vi "FindAndHighlightPoint.vi"(7 "Data In":T1={"Calibration Input"=[], "CalibrationResults"={"Center in Pixels"=[374.0120339529387, 375.46592887074246], "Angle"=0.022945275255000355, "Pixels/MHz X"=0.0, "Pixels/MHz Y"=0.0}, "Highlight"=[], "Running Script"=refnum}, 8 "error in (no error)":errorcluster, 9 "Vertical":i32, 10 "Horizontal":i32, 11 "Value":i32[][](array[numeric])) -> (0 "error out":errorcluster, 2 "Data Out":T1={"Calibration Input"=[], "CalibrationResults"={"Center in Pixels"=[374.0120339529387, 375.46592887074246], "Angle"=0.022945275255000355, "Pixels/MHz X"=0.0, "Pixels/MHz Y"=0.0}, "Highlight"=[], "Running Script"=refnum}, 3 "Numeric":i32)   [LabVIEW 2017]
uses:
  TypeDefinitions/ExperimentVariables.ctl
  ImageAcquisitionProgram/ImageAcquisitionLibrary/GlobalFrontPanelReferences.vi
  ImageAcquisitionProgram/ImageAcquisitionLibrary/ImageAcquisitionLibrary.lvlib
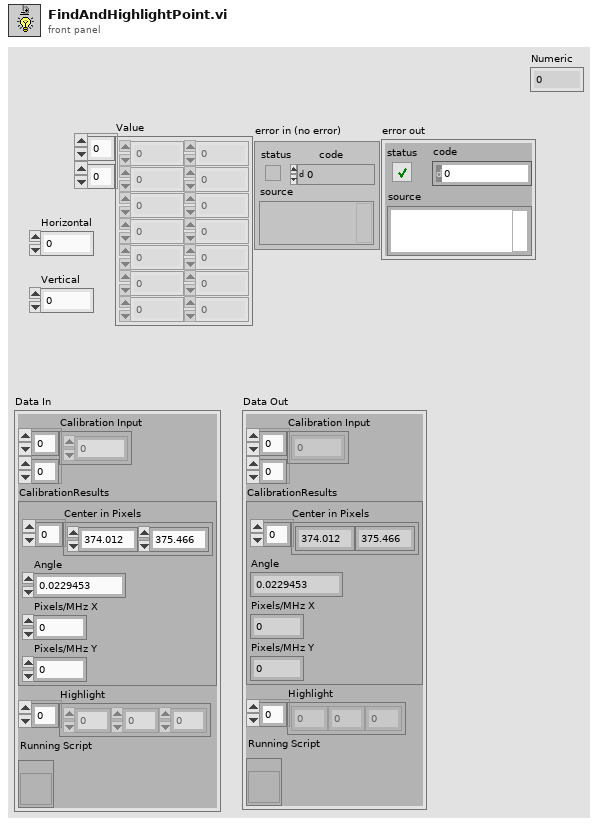
[diagram p1: front panel]
types:
  T1 = typedef "ExperimentVariables.ctl" = cluster{"Calibration Input":i32[][], "CalibrationResults":cluster{"Center in Pixels":dbl[], "Angle":dbl, "Pixels/MHz X":dbl, "Pixels/MHz Y":dbl}, "Highlight":i32[], "Running Script":refnum<vi>}
  T2 = typedef "ImageAcquisitionLibrary.lvlib/MarkersArray.ctl" = T3[]
  T3 = typedef "ImageAcquisitionLibrary.lvlib/Marker.ctl" = cluster{"X":dbl, "Color":u32, "Y ":dbl, "Owner":u8}
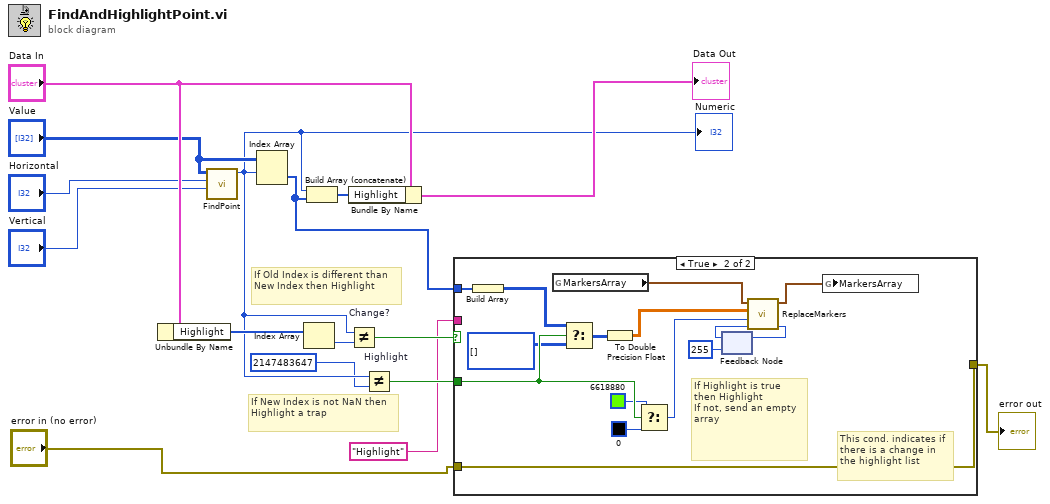
[diagram p0: block diagram]
diagram:
  # "If New Index is not NaN then Highlight a trap"
  # "If Old Index is different than New Index then Highlight"
  n1 = Unbundle By Name("Data In") -> ("Highlight"=w11:i32[])
  n2 = call "FindPoint.vi"("Vertical"="Vertical", "Horizontal"="Horizontal", "Value"="Value") -> ("Numeric"=w7:i32)  [unwired: 8 in]
  "Numeric" <- w7
  n3 = Index Array(array="Value", index (row)=w7) -> (element=w4:i32[])  [unwired: 1 in]
  n4 = Index Array(array=w11) -> (element=w10:i32)  [unwired: 1 in]
  n5 = Build Array (concatenate)(w7, w4) -> (w14:i32[])
  n6 = Bundle By Name(cluster="Data In", "Highlight"=w14) -> (→"Data Out":T1)
  n7 = Not Equal? "Change?"(x=w7, y=w10) -> (x != y?=w9:bool)
  n8 = Not Equal? "Highlight"(x=w7, y=2147483647) -> (x != y?=w6:bool)
  n9 = case shown="True" w9 {
    tunnel: w6 -> [_ w29]
    tunnel: w4 -> [_ w32]
    tunnel: "Highlight" ("Group") -> [_ _]
    tunnel: [w17 w28] -> w3
    tunnel: "error in (no error)" -> [w17 w28]
    frame False {
    }
    frame True {
      # "If Highlight is true then Highlight\nIf not, send an empty array"
      # "This cond. indicates if there is a change in the highlight list"
      n10 = Build Array(w32) -> (w26:i32[][])
      n11 = global read "GlobalFrontPanelReferences.vi" "MarkersArray"() -> (w24:T2)
      n12 = Select(t=w26, s=w29, f=i32[][] []) -> (s? t:f=w19:i32[][])
      n13 = To Double Precision Float(number=w19) -> (double precision float=w18:dbl[][])
      n14 = Select(t=u32 6618880 ("Color"), s=w29, f=u32 0 ("Color")) -> (s? t:f=w22:u32)
      n15 = feedback #1(u8 255 ("Owner Out")) -> (w21:u8)
      n16 = call "ReplaceMarkers.vi"("Owner"=w21, "Color"=w22, "Pixels 3"=w18, "MarkersArray"=w24) -> ("Owner Out"=w20:u8, "MarkersArray Out"=w23:T2)  [unwired: 6 in]
      n17 = feedback-in #1(w20) -> ()
      n18 = global write "GlobalFrontPanelReferences.vi" "MarkersArray"(w23) -> ()
    }
  }
  "error out" <- w3
